vi "AutoCheckHotGoal.vi"(7 "HotGoalType":T1, 8 "error in (no error)":errorcluster, 9 "PreCheckGoalWait":u32, 10 "AutoMode":T2, 11 "CheckHotGoalTimeout":u32=800) -> (0 "error out":errorcluster, 2 "CheckGoalTimedOut?":bool, 3 "Hot?":bool)   [LabVIEW 2013]
uses:
  AutoMode.ctl
  HotGoalDetectType.ctl
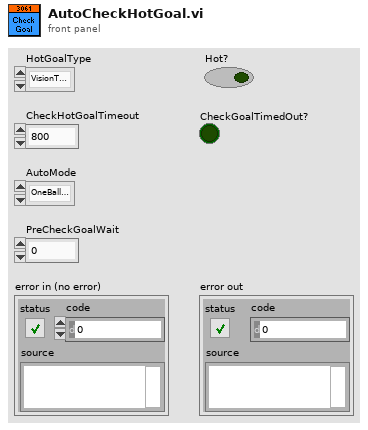
[diagram p1: front panel]
types:
  T1 = typedef "HotGoalDetectType.ctl" = enum16{"VisionTarget", "Kinect", "SoundDetect", "Webcam"}
  T2 = typedef "AutoMode.ctl" = enum16{"OneBallFront", "OneBallCollector", "TwoBallNormal", "TwoBallHot"}
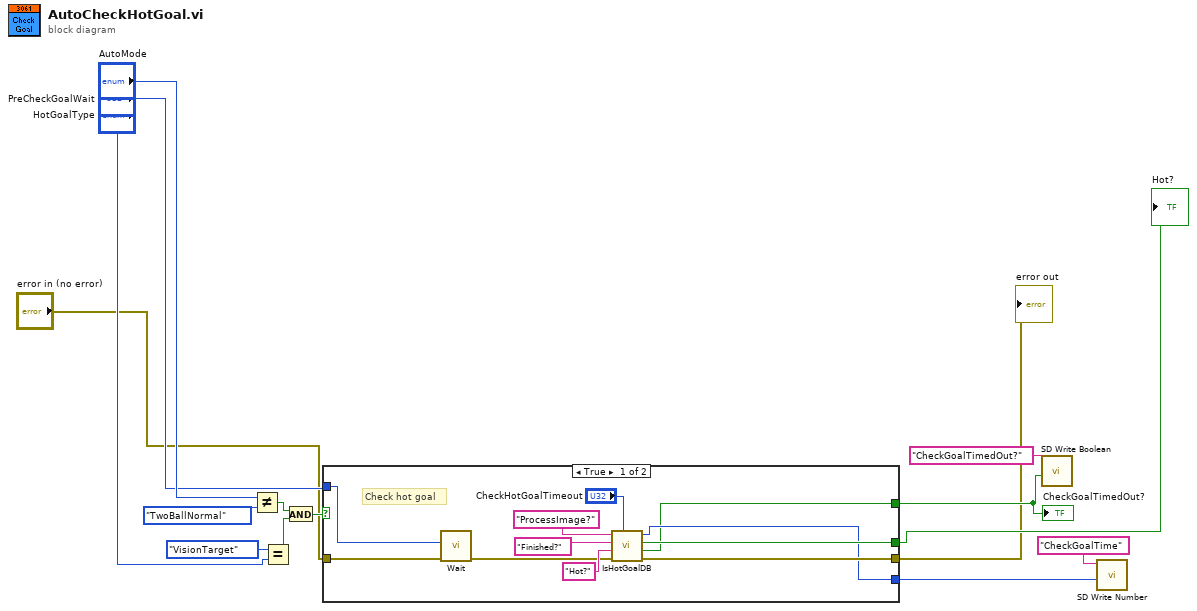
[diagram p0: block diagram]
diagram:
  n1 = Not Equal?(x="AutoMode", y=AutoMode."TwoBallNormal") -> (x != y?=w11:bool)
  n2 = Equal?(x=HotGoalDetectType."VisionTarget", y="HotGoalType") -> (x = y?=w9:bool)
  n3 = And(x=w11, y=w9) -> (x .and. y?=w10:bool)
  n4 = case shown="True" w10 {
    tunnel: "error in (no error)" -> [w22 w27]
    tunnel: [w21 w27] -> w2
    tunnel: [w18 _] -> w3
    tunnel: "PreCheckGoalWait" -> [w19 _]
    tunnel: [w17 _] -> w6
    tunnel: [w16 _] -> w7
    frame True {
      # "Check hot goal"
      n5 = call "Wait.vi"("error in"=w22, "milliseconds to wait"=w19) -> ("error out"=w20:errorcluster)  [unwired: 9 in]
      n6 = call "IsHotGoalDB.vi"("Timeout (ms)"="CheckHotGoalTimeout", "error in"=w20, "DBHot?"="Hot?", "DBFinished?"="Finished?", "DBStart"="ProcessImage?") -> ("error out"=w21:errorcluster, "TimedOut?"=w16:bool, "Hot?"=w18:bool, "ElapsedTime"=w17:u32)  [unwired: 3 in]
    }
    frame False {
    }
  }
  "CheckGoalTimedOut?" <- w7
  "Hot?" <- w3
  "error out" <- w2
  n7 = call <vilib>:"SD Write Boolean.vi"("Boolean"=w7, "Name"="CheckGoalTimedOut?") -> ()  [unwired: 8 in, 2 out]
  n8 = call <vilib>:"SD Write Number.vi"("Numeric"=w6, "Name"="CheckGoalTime") -> ()  [unwired: 8 in, 2 out]
